vi "test_libssh2_session_block_directions.vi"() -> ()   [LabVIEW 2013, in "libssh2_integration_tests.lvlib"]
uses:
  libssh2_integration_tests.lvlib
  libssh2/libssh2_session_block_direction.ctl
  <vilib>/addons/_JKI Toolkits/Caraya/classes/Test/Test.lvclass
  support/support.lvlib
  libssh2/libssh2.lvlib
  <vilib>/addons/_JKI Toolkits/Caraya/classes/Assert/Assert.lvclass
panel:
  out "error out":errorcluster
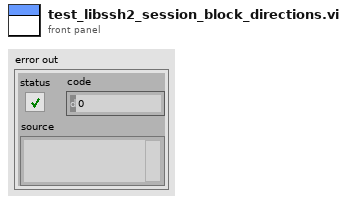
[diagram p1: front panel]
types:
  T1 = typedef "libssh2.lvlib/Session Refnum.ctl" = refnum<k1>
  T2 = typedef "libssh2.lvlib/Channel Refnum.ctl" = refnum<k1>
  T3 = typedef "libssh2.lvlib/libssh2_session_block_direction.ctl" = i32
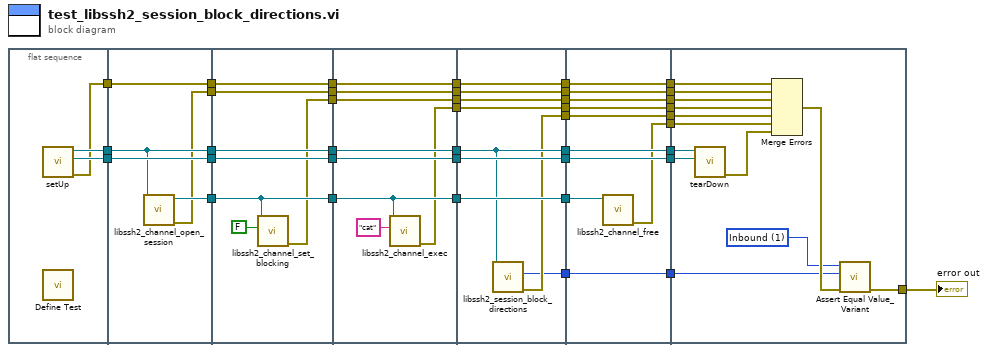
[diagram p0: block diagram]
diagram:
  n1 = flat-sequence {
    tunnel: [w43] -> w40
    tunnel: [w42] -> w39
    tunnel: [w41] -> w38
    tunnel: w40 -> [w47]
    tunnel: w39 -> [w48]
    tunnel: [w47] -> w30
    tunnel: [w48] -> w28
    tunnel: [w46] -> w22
    tunnel: w38 -> [w45]
    tunnel: [w45] -> w26
    tunnel: [w44] -> w24
    tunnel: w30 -> [w55]
    tunnel: [w55] -> w29
    tunnel: w28 -> [w54]
    tunnel: [w54] -> w27
    tunnel: w26 -> [w53]
    tunnel: [w53] -> w25
    tunnel: w24 -> [w52]
    tunnel: [w52] -> w23
    tunnel: w22 -> [w51]
    tunnel: [w51] -> w21
    tunnel: [w49] -> w20
    tunnel: w29 -> [w63]
    tunnel: [w63] -> w18
    tunnel: w27 -> [w62]
    tunnel: [w62] -> w17
    tunnel: w25 -> [w61]
    tunnel: [w61] -> w16
    tunnel: w23 -> [w60]
    tunnel: [w60] -> w15
    tunnel: w21 -> [w59]
    tunnel: [w59] -> w14
    tunnel: [w57] -> w13
    tunnel: w20 -> [w56]
    tunnel: [w56] -> w12
    tunnel: w18 -> [w66]
    tunnel: [w66] -> w10
    tunnel: w17 -> [w72]
    tunnel: [w72] -> w9
    tunnel: w16 -> [w71]
    tunnel: [w71] -> w8
    tunnel: w15 -> [w70]
    tunnel: [w70] -> w7
    tunnel: w14 -> [w67]
    tunnel: [w67] -> w6
    tunnel: w13 -> [w69]
    tunnel: [w69] -> w5
    tunnel: w12 -> [w68]
    tunnel: [w68] -> w4
    tunnel: [w65] -> w3
    tunnel: [w64] -> w2
    tunnel: w10 -> [w82]
    tunnel: w9 -> [w81]
    tunnel: [w82] -> w37
    tunnel: [w81] -> w36
    tunnel: [w80] -> w35
    tunnel: w8 -> [w79]
    tunnel: [w79] -> w34
    tunnel: w7 -> [w78]
    tunnel: [w78] -> w33
    tunnel: w6 -> [w77]
    tunnel: w5 -> [w76]
    tunnel: [w76] -> w31
    tunnel: w4 -> [w75]
    tunnel: [w75] -> w19
    tunnel: w3 -> [w74]
    tunnel: [w74] -> w11
    tunnel: w2 -> [w73]
    tunnel: [w73] -> w1
    tunnel: w37 -> [w95]
    tunnel: w36 -> [w94]
    tunnel: [w93] -> w32
    tunnel: w35 -> [w91]
    tunnel: w34 -> [w90]
    tunnel: w33 -> [w88]
    tunnel: w31 -> [w87]
    tunnel: w19 -> [w86]
    tunnel: w11 -> [w85]
    tunnel: w1 -> [w84]
    frame #0 {
      n2 = call "setUp.vi"() -> ("error out"=w41:errorcluster, "connection ID"=w42:refnum<k5>, "session"=w43:T1)  [unwired: 9 in]
      n3 = call <vilib>:"Define Test.vi"() -> ()  [unwired: 10 in, 2 out]
    }
    frame #1 {
      n4 = call "libssh2_channel_open_session.vi"("session"=w47) -> ("error out"=w44:errorcluster, "channel"=w46:T2)  [unwired: 9 in]
    }
    frame #2 {
      n5 = call "libssh2_channel_set_blocking.vi"("blocking"=FALSE, "channel"=w51) -> ("error out"=w49:errorcluster)  [unwired: 9 in]
    }
    frame #3 {
      n6 = call "libssh2_channel_exec.vi"("command"="cat", "channel"=w59) -> ("error out"=w57:errorcluster)  [unwired: 9 in]
    }
    frame #4 {
      n7 = call "libssh2_session_block_directions.vi"("session"=w66) -> ("error out"=w65:errorcluster, "block direction"=w64:T3)  [unwired: 9 in]
    }
    frame #5 {
      n8 = call "libssh2_channel_free.vi"("channel"=w77) -> ("error out"=w80:errorcluster)  [unwired: 10 in]
    }
    frame #6 {
      w83 = T3 1 items=["Inbound"=1, "Outbound"=2] ("block direction")
      n9 = call "tearDown.vi"("connection ID"=w94, "session"=w95) -> ("error out"=w92:errorcluster)  [unwired: 9 in]
      n10 = Merge Errors(w90, w88, w86, w87, w85, w91, w92) -> (w89:errorcluster)
      n11 = call <vilib>:"Assert Equal Value_Variant.vi"("error in (no error)"=w89, "Y"=w84, "X"=w83) -> ("error out"=w93:errorcluster)  [unwired: 7 in, 1 out]
    }
  }
  "error out" <- w32
